vi "sub_waypoint_load.vi"(11 "path":path) -> (2 "stop pt":cluster{"x":dbl, "y":dbl}[](array[cluster]), 3 "way pt":cluster{"X":dbl, "Y":dbl}[](graph))   [LabVIEW 2019]
uses:
  Ctrl/cmd_common.ctl
panel:
  out "name":string
  out "n":i32
  out "read":string
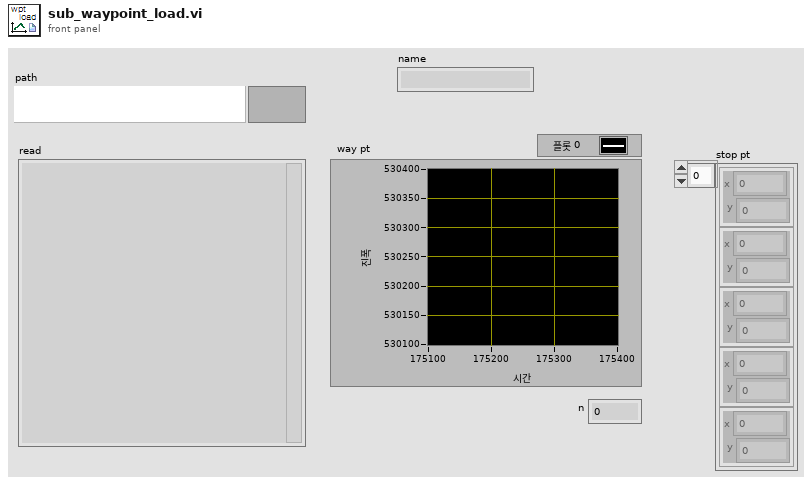
[diagram p1: front panel]
types:
  T1 = typedef "cmd_common.ctl" = enum16{"read", "write"}
  T2 = cluster{"배열 타입(2D Dbl)[0]":dbl, "배열 타입(2D Dbl)[1]":dbl}[]
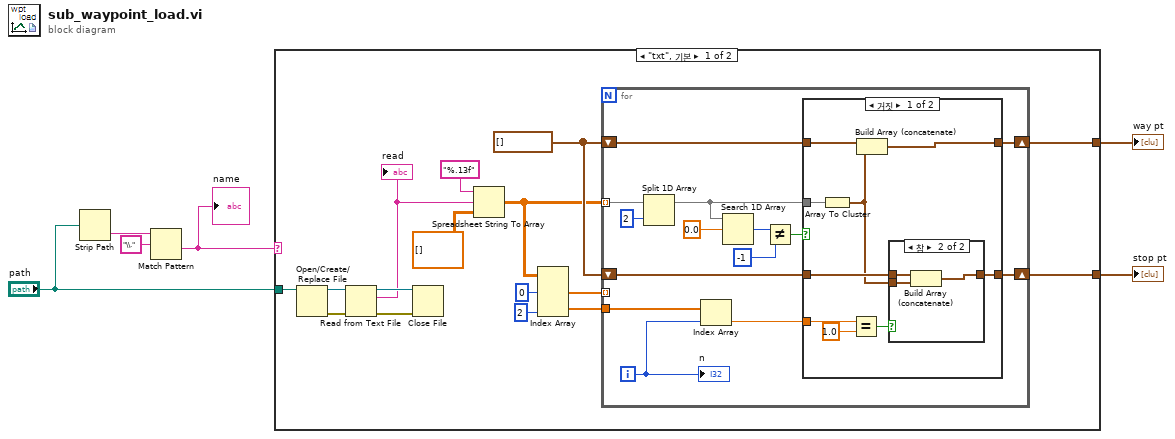
[diagram p0: block diagram]
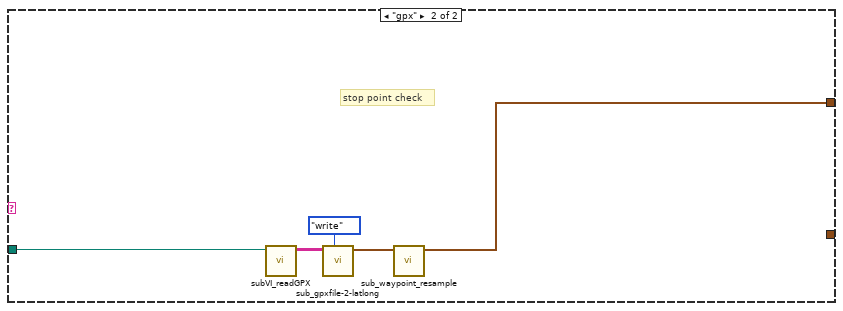
[diagram p4: hidden frame]
diagram:
  n1 = Strip Path(path="path") -> (name=w4:string)  [unwired: 1 out]
  n2 = Match Pattern(string=w4, regular expression="\\.") -> (after substring=w1:string)  [unwired: 1 in, 3 out]
  "name" <- w1
  n3 = case shown="\"txt\", 기본" w1 {
    tunnel: [w19 w52] -> w6
    tunnel: [w15 _] -> w5
    tunnel: "path" -> [w12 w54]
    frame "txt", Default {
      w18 = T2 []
      n4 = Open/Create/Replace File(file path (use dialog)=w12) -> (refnum out=w14:refnum<file>, error out=w10:errorcluster)  [unwired: 5 in, 1 out]
      n5 = Read from Text File(file (use dialog)=w14, error in=w10) -> (refnum out=w13:refnum<file>, text=w11:string, error out=w9:errorcluster)  [unwired: 2 in, 1 out]
      "read" <- w11
      n6 = Close File(refnum=w13, error in=w9) -> ()  [unwired: 2 out]
      n7 = Spreadsheet String To Array(format string="%.13f" ("포맷 문자열"), spreadsheet string=w11, array type (2D Dbl)=dbl[][] [] ("배열 타입(2D Dbl)")) -> (array=w16:dbl[][])  [unwired: 1 in]
      n8 = Index Array(array=w16, index (col) #1=0 ("비활성화된 인덱스 (열)"), index (col) #2=2 ("indx")) -> (element #1=w7:dbl[], element #2=w17:dbl[])  [unwired: 2 in]
      n9 = for {
        tunnel: w16 -> [w31] mode=indexing
        shift-right: [w36] -> w19
        shift-left: w18 -> [w35]
        shift-right: [w32] -> w15
        shift-left: w18 -> [w33]
        tunnel: w17 -> [w25]
        tunnel: w7 -> [_] mode=indexing
        i -> [w24]
        n10 = Split 1D Array(array=w31, index=2 ("인덱스")) -> (first subarray=w30:dbl[])  [unwired: 1 out]
        n11 = Index Array(array=w25, index=w24) -> (element=w23:dbl)
        n12 = Search 1D Array(1D array=w30, element=0.0 ("원소")) -> (index of element=w28:i32)  [unwired: 1 in]
        n13 = Not Equal?(x=w28, y=-1) -> (x != y?=w26:bool)
        n14 = case shown="거짓" w26 {
          tunnel: [w45 w51] -> w36
          tunnel: w35 -> [w44 w51]
          tunnel: w30 -> [w43 _]
          tunnel: w33 -> [w40 w50]
          tunnel: w23 -> [w39 _]
          tunnel: [w38 w50] -> w32
          frame False {
            n15 = Array To Cluster(array=w43) -> (cluster=w37:cluster{"[0]":dbl, "[1]":dbl})
            n16 = Equal?(x=w39, y=1.0) -> (x = y?=w42:bool)
            n17 = Build Array (concatenate)(w44, w37) -> (w45:cluster{"[0]":dbl, "[1]":dbl}[])
            n18 = case shown="참" w42 {
              tunnel: w40 -> [w46 w49]
              tunnel: [w46 w48] -> w38
              tunnel: w37 -> [_ w47]
              frame False {
              }
              frame True {
                n19 = Build Array (concatenate)(w49, w47) -> (w48:cluster{"[0]":dbl, "[1]":dbl}[])
              }
            }
          }
          frame True {
            # "0,0 waypoint del"
          }
        }
        "n" <- w24
      }
    }
    frame "gpx" {
      # "stop point check"
      n20 = call "subVI_readGPX.vi"("path"=w54) -> ("wpt Array"=w56:string[][])  [unwired: 8 in]
      n21 = call "sub_gpxfile-2-latlong.vi"("cmd"=cmd_common."write", "wpt Array"=w56) -> ("tm"=w53:cluster{dbl, dbl}[])  [unwired: 8 in, 1 out]
      n22 = call "sub_waypoint_resample.vi"("line point"=w53) -> ("interpolate 1d array"=w52:cluster{dbl, dbl}[])  [unwired: 9 in, 1 out]
    }
  }
  "way pt" <- w6
  "stop pt" <- w5
